vi "Format App Version String.vi"(3 "App Version String in":string) -> (1 "App Version String":string)   [LabVIEW 2020, in "Builder Core.lvlib"]
uses:
  Builder Core.lvlib
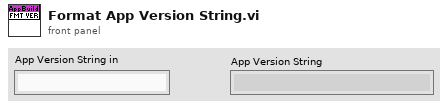
[diagram p1: front panel]
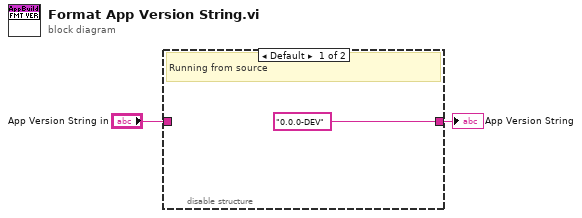
[diagram p0: block diagram]
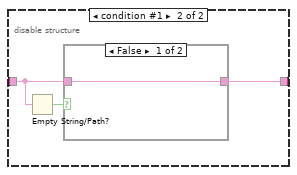
[diagram p2: hidden frame]
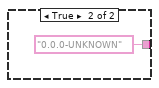
[diagram p3: hidden frame]
diagram:
  n1 = disable-structure shown="Default" {
    disable-tunnel: "App Version String in" -> [_ w5]
    disable-tunnel: ["0.0.0-DEV" ("Version String") w4] -> w1
    frame condition #0 (active) {
      # "Running from source"
    }
    frame condition #1 {
      n2 = Empty String/Path?(string/path=w5) -> (empty?=w6:bool)
      n3 = case shown="False" w6 {
        tunnel: w5 -> [w7 _]
        tunnel: [w7 "0.0.0-UNKNOWN" ("Version String in")] -> w4
        frame False {
        }
        frame True {
        }
      }
    }
  }
  "App Version String" <- w1
